vi "5.6.vi"() -> ()   [LabVIEW 2017]
uses:
  <vilib>/measure/NI_MABase.lvlib
panel:
  out "大小":i32
  out "最大值":dbl
  out "Y":dbl[](array[numeric])
  out "dt":dbl
  in  "sampling info":cluster{"Fs":dbl, "#s":dbl}={"Fs"=1000.0, "#s"=1000.0} caption="采样信息" {"Fs" format="%.2p"}
  in  "相位":dbl format="%.2p"
  in  "幅值":dbl=1.0 format="%0.2p"
  in  "频率":dbl=10.0 format="%0.2p"
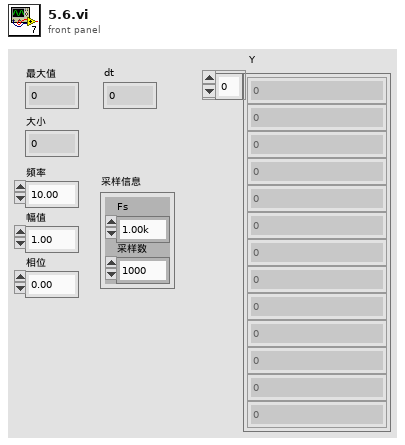
[diagram p1: front panel]
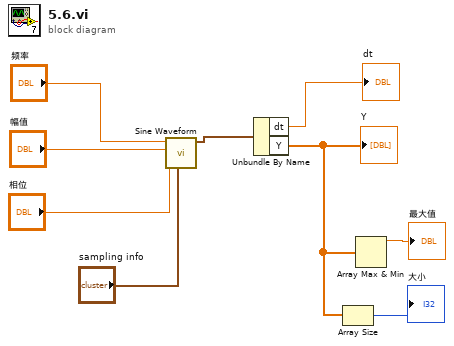
[diagram p0: block diagram]
diagram:
  n1 = call <vilib>:"Sine Waveform.vi"("sampling info"="sampling info", "phase"="相位", "amplitude"="幅值", "frequency"="频率") -> ("signal out"=w5:waveform(dbl))  [unwired: 6 in, 1 out]
  n2 = Unbundle By Name(w5) -> ("dt"=→"dt":dbl, "Y"=w1:dbl[])
  "Y" <- w1
  n3 = Array Size(array=w1) -> (size(s)=→"大小":i32)
  n4 = Array Max & Min(array=w1) -> (max value=→"最大值":dbl)  [unwired: 3 out]
